vi "Open XML Configuration From File.vi"(6 "XML Schema File Path":path=path "C:/Program Files (x86)/National Instruments/LabVIEW 2020/instr.lib/BTICardLib/XML Schema/BTI.xsd", 8 "error in":errorcluster, 9 "Validate Schema (F)":bool, 11 "XML Configuration File Path":path=path "E:/Ballard - Arinc-429 CD/Example Database/Ballard/XML_000.XML") -> (0 "error out":errorcluster, 1 "schemaVersion":i32, 2 "name":string, 3 "xml ref out":refnum<k24>)   [LabVIEW 2020, in "Ballard_1553_Hardware_ni.lvlib"]
uses:
  Ballard_1553_Hardware_ni.lvlib
  C:/Users/Administrator/Desktop/GIT/Ballard-MIL-STD-1553-Custom-Device/Source/System Explorer/SubVIs/Parse XML Ballard/1.2/BTIXML_SerDes.dll
  Ballard-MIL-STD-1553-Custom-Device/Source/System Explorer/SubVIs/Parse XML Ballard/1.2/BTIXML_SerDes.dll
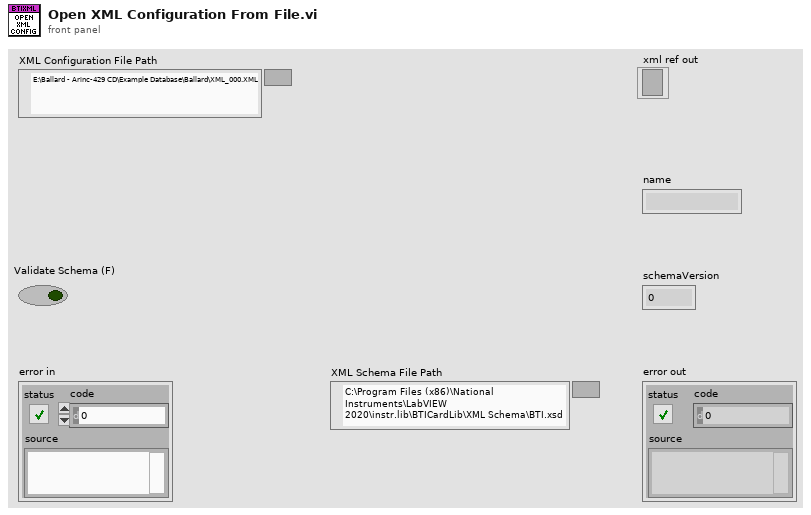
[diagram p1: front panel]
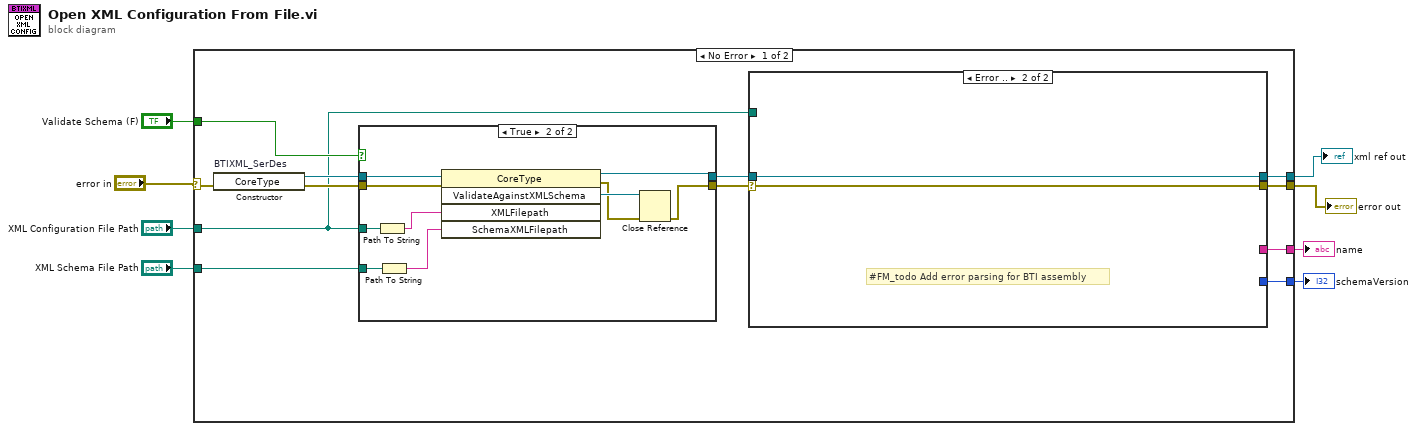
[diagram p0: block diagram]
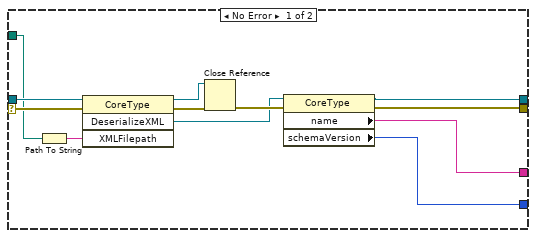
[diagram p2: hidden frame]
diagram:
  n1 = case shown="No Error" "error in" {
    selector: "error in" -> [w17 w47]
    tunnel: "Validate Schema (F)" -> [w19 _]
    tunnel: "XML Configuration File Path" -> [w11 _]
    tunnel: "XML Schema File Path" -> [w16 _]
    tunnel: [w13 w47] -> w4
    tunnel: [w12 _] -> w3
    tunnel: [w10 _] -> w2
    tunnel: [w9 _] -> w1
    frame No Error {
      n2 = constructor on="BTIXML_SerDes" class="CoreType"(error in=w17) -> (reference out=w18:refnum<k24>, error out=w20:errorcluster)  [unwired: 2 in, 1 out]
      n3 = case shown="True" w19 {
        tunnel: w20 -> [w36 w45]
        tunnel: w18 -> [w35 w46]
        tunnel: w11 -> [_ w44]
        tunnel: w16 -> [_ w43]
        tunnel: [w36 w38] -> w14
        tunnel: [w35 w37] -> w15
        frame False {
        }
        frame True {
          n4 = Path To String(path=w44) -> (string=w41:string)
          n5 = Path To String(path=w43) -> (string=w42:string)
          n6 = invoke class="CoreType" method="ValidateAgainstXMLSchema"(reference=w46, error in=w45, "XMLFilepath"=w41, "SchemaXMLFilepath"=w42) -> (reference out=w37:refnum<k24>, error out=w39:errorcluster, "ValidateAgainstXMLSchema"=w40:refnum<k24>)  [unwired: 1 in, 2 out]
          n7 = Close Reference(reference=w40, error in (no error)=w39) -> (error out=w38:errorcluster)
        }
      }
      n8 = case shown="Error .." w14 {
        selector: w14 -> [w31 w34]
        tunnel: w15 -> [w32 w33]
        tunnel: [w24 w34] -> w13
        tunnel: [w23 w33] -> w12
        tunnel: w11 -> [w29 _]
        tunnel: [w22 _] -> w10
        tunnel: [w21 _] -> w9
        frame No Error {
          n9 = Path To String(path=w29) -> (string=w30:string)
          n10 = invoke class="CoreType" method="DeserializeXML"(reference=w32, error in=w31, "XMLFilepath"=w30) -> (reference out=w27:refnum<k24>, error out=w28:errorcluster, "DeserializeXML"=w25:refnum<k24>)  [unwired: 1 in, 1 out]
          n11 = Close Reference(reference=w27, error in (no error)=w28) -> (error out=w26:errorcluster)
          n12 = property class="CoreType"(reference=w25, error in=w26) -> (reference out=w23:refnum<k24>, error out=w24:errorcluster, "name"=w22:string, "schemaVersion"=w21:i32)
        }
        frame Error {
          # "#FM_todo Add error parsing for BTI assembly"
        }
      }
    }
    frame Error {
    }
  }
  "error out" <- w4
  "xml ref out" <- w3
  "name" <- w2
  "schemaVersion" <- w1
